vi "Read Location in range.vi"(9 "Read Size":u32, 10 "Circular Buffer Size":u32, 11 "Read Location":i32) -> (2 "Corrected Read Size":u32, 3 "Corrected Read Locaton":u32)   [LabVIEW 2023]
doc: "Author: Scott Hannahs <sth@magnet.fsu.edu>\nCopyright 2018 Florida State University, All rights reserved."
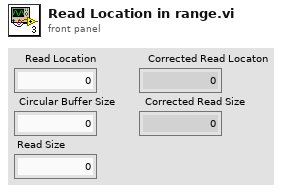
[diagram p1: front panel]
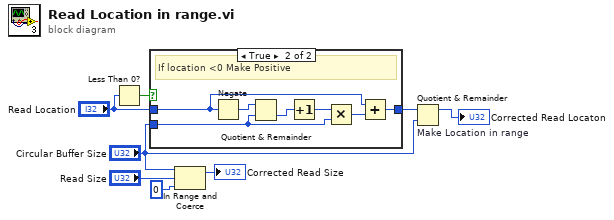
[diagram p0: block diagram]
diagram:
  n1 = Less Than 0?(x="Read Location") -> (x < 0?=w5:bool)
  n2 = case shown="True" w5 {
    tunnel: "Circular Buffer Size" -> [_ w13]
    tunnel: "Read Location" -> [w9 w11]
    tunnel: [w9 w10] -> w7
    frame False {
      # "Location is Positive"
    }
    frame True {
      # "If location <0 Make Positive"
      n3 = Negate(x=w11) -> (-x=w16:i32)
      n4 = Quotient & Remainder(x=w16, y=w13) -> (floor(x/y)=w15:u32)  [unwired: 1 out]
      n5 = Increment(x=w15) -> (x+1=w14:u32)
      n6 = Multiply(x=w14, y=w13) -> (x*y=w12:u32)
      n7 = Add(x=w11, y=w12) -> (x+y=w10:u32)
    }
  }
  n8 = In Range and Coerce(upper limit="Circular Buffer Size", x="Read Size", lower limit=u32 0) -> (coerced(x)=→"Corrected Read Size":u32)  [unwired: 1 out]
  n9 = Quotient & Remainder "Make Location in range"(x=w7, y="Circular Buffer Size") -> (x-y*floor(x/y)=→"Corrected Read Locaton":u32)  [unwired: 1 out]
